vi "Poly Set Map Build.vi"(10 "Poly Ref":refnum<vi>, 11 "Poly Set Map in":T1) -> (3 "Poly Set Map out":T1)   [LabVIEW 2020]
uses:
  _td_cluster_InstanceInfo.ctl
  _td_map_PolyInstanceInfo.ctl
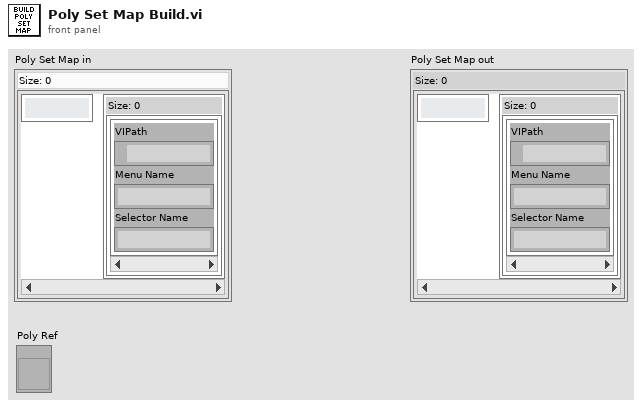
[diagram p1: front panel]
types:
  T1 = typedef "_td_map_PolyInstanceInfo.ctl" = map{string, set{T2}}
  T2 = typedef "_td_cluster_InstanceInfo.ctl" = cluster{"VIPath":path, "Menu Name":string, "Selector Name":string}
  T3 = cluster{"VIPath":path, "Menu Name":string, "Selector Name":string}[]
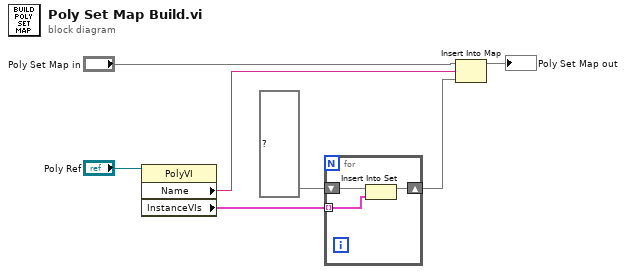
[diagram p0: block diagram]
diagram:
  n1 = property class="PolyVI"(reference="Poly Ref") -> ("Name"=w6:string, "InstanceVIs"=w5:T3)  [unwired: 1 in, 2 out]
  n2 = for {
    shift-right: [w10] -> w4
    shift-left: set{T2} {} ("value") -> [w9]
    tunnel: w5 -> [w8] mode=indexing
    n3 = Insert Into Set(10:w8, 11:w9) -> (3:w10:set{T2})  [unwired: 1 out]
  }
  n4 = Insert Into Map(map in="Poly Set Map in", key=w6, value=w4) -> (map out=→"Poly Set Map out":T1)  [unwired: 2 out]
